vi "nrs.sunrise-time-table.vi"() -> (1 "Irrigation Timing":T1, 2 "Sunrise Timing":cluster{"Sunset":timestamp, "Sunrise":timestamp}, 3 "Solar Elevation Graph":waveform(dbl))   [LabVIEW 2024]
uses:
  globals/globals-engine.vi
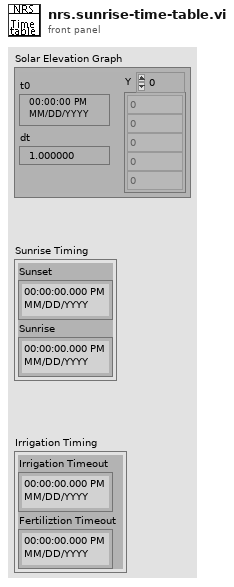
[diagram p1: front panel]
types:
  T1 = cluster{"Irrigation Timeout":timestamp, "Fertiliztion Timeout":timestamp}
  T2 = typedef "irr-panel.ctl" = cluster{"Day Time":cluster{"Sunset":timestamp, "Sunrise":timestamp}, "timeLimits":cluster{"Irrigation":dbl, "Nut./Water":dbl}, "Calculated Timing":cluster{"Irrigation Timeout":timestamp, "Nutrients Timeout":timestamp}, "Irr Dosing Time":cluster{"Nutrients":u16, "Water":u16, "Wash":u16}, "UV Limit ":dbl, "Dose Table":cluster{"Enable":bool, "output":string}[], "Last Iteration":timestamp, "UV Reduction Status":bool, "UV Reduction":u8}
  T3 = typedef "type.eng.settings.ctl" = cluster{"Project Name":string, "Latitude":dbl, "Longitude":dbl, "TimeZone":i32, "userName":string}
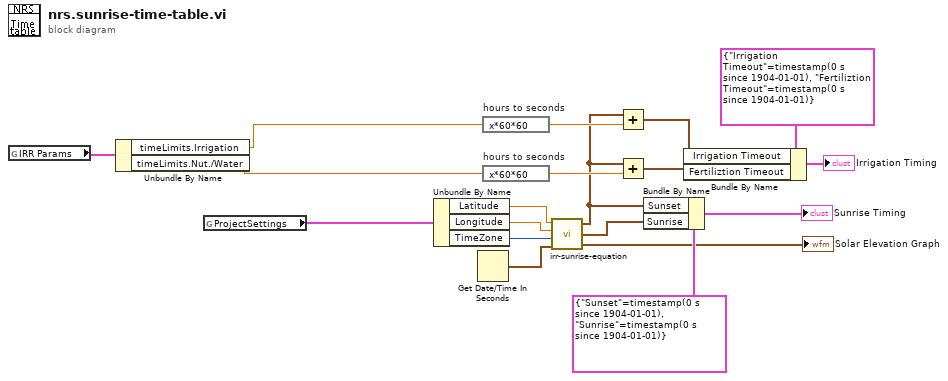
[diagram p0: block diagram]
diagram:
  n1 = global read "globals-engine.vi" "IRR Params"() -> (w4:T2)
  n2 = Unbundle By Name(w4) -> ("timeLimits.Irrigation"=w10:dbl, "timeLimits.Nut./Water"=w12:dbl)
  n3 = global read "globals-engine.vi" "ProjectSettings"() -> (w8:T3)
  n4 = Unbundle By Name(w8) -> ("Latitude"=w7:dbl, "Longitude"=w6:dbl, "TimeZone"=w5:i32)
  n5 = Get Date/Time In Seconds() -> (seconds since 1Jan1904=w9:timestamp)
  n6 = expression code="x*60*60" "hours to seconds"(w10) -> (w11:dbl)
  n7 = expression code="x*60*60" "hours to seconds"(w12) -> (w13:dbl)
  n8 = call "irr-sunrise-equation.vi"("Date"=w9, "Time Zone (+ to E)"=w5, "Longitude (+ to E)"=w6, "Latitude (+ to N)"=w7) -> ("Solar Elevation Graph"=→"Solar Elevation Graph":waveform(dbl), "Sunrise (LST)"=w19:timestamp, "Sunset (LST)"=w3:timestamp)
  n9 = Add(x=w3, y=w11) -> (x+y=w2:timestamp)
  n10 = Add(x=w3, y=w13) -> (x+y=w1:timestamp)
  n11 = Bundle By Name(cluster=cluster{"Sunset":timestamp, "Sunrise":timestamp} {"Sunset"=timestamp(0 s since 1904-01-01), "Sunrise"=timestamp(0 s since 1904-01-01)} ("Cluster 3"), "Sunset"=w3, "Sunrise"=w19) -> (→"Sunrise Timing":cluster{"Sunset":timestamp, "Sunrise":timestamp})
  n12 = Bundle By Name(cluster=T1 {"Irrigation Timeout"=timestamp(0 s since 1904-01-01), "Fertiliztion Timeout"=timestamp(0 s since 1904-01-01)} ("Cluster 2"), "Irrigation Timeout"=w2, "Fertiliztion Timeout"=w1) -> (→"Irrigation Timing":T1)
